vi "Export Properties.vi"(8 "error in (no error)":errorcluster, 10 "Properties":T1[](array[typedef]), 11 "Node in":refnum<k20>) -> (0 "error out":errorcluster, 3 "Node out":refnum<k20>)   [LabVIEW 2013, in "JUnit for Azure Pipelines.lvclass"]
uses:
  JUnit for Azure Pipelines.lvclass
  Test Case Property.ctl
  <vilib>/xml/Close Reference(Node).vi
  <vilib>/xml/NI_XML.lvlib
  XML/XML.lvlib
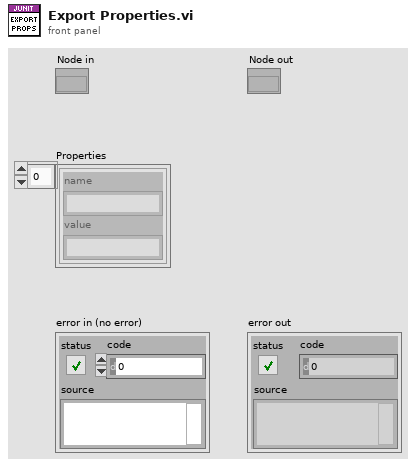
[diagram p1: front panel]
types:
  T1 = typedef "JUnit for Azure Pipelines.lvclass/Test Case Property.ctl" = cluster{"name":string, "value":string}
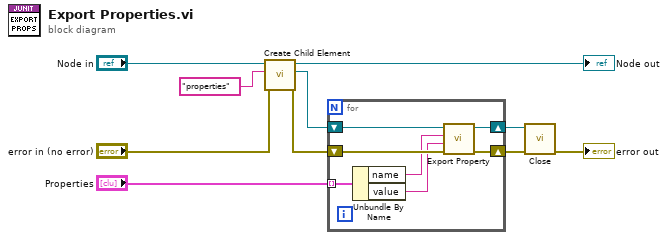
[diagram p0: block diagram]
diagram:
  n1 = call "Create Child Element.vi"("error in (no error)"="error in (no error)", "Name"="properties" ("Tag Name"), "Element in"="Node in") -> ("error out"=w5:errorcluster, "Child Element"=w4:refnum<k20>, "Element out"=→"Node out":refnum<k20>)  [unwired: 6 in]
  n2 = for {
    shift-right: [w16] -> w2
    shift-left: w4 -> [w17]
    shift-right: [w15] -> w1
    shift-left: w5 -> [w14]
    tunnel: "Properties" -> [w13] mode=indexing
    n3 = Unbundle By Name(w13) -> ("name"=w12:string, "value"=w11:string)
    n4 = call "Export Property.vi"("error in (no error)"=w14, "Value"=w11, "Name"=w12, "Node in"=w17) -> ("error out"=w15:errorcluster, "Node out"=w16:refnum<k20>)  [unwired: 6 in]
  }
  n5 = call-poly <vilib>:"Close.vi"("error in (no error)"=w1, "node"=w2) -> ("error out"=→"error out":errorcluster)  [unwired: 7 in]
